vi "Update Connection.vi"(8 "error in (no error)":errorcluster, 10 "Connection Info":T1, 11 "VectoService in":refnum<class "VectoInfo.lvclass">) -> (0 "error out":errorcluster, 3 "VectoService out":refnum<class "VectoInfo.lvclass">)   [LabVIEW 2020, in "Vecto.lvlib" / "VectoInfo.lvclass"]
uses:
  VectoInfo.lvclass
  Connection Info.ctl
  Connection Type.ctl
  Connection Data.ctl
  VectoInfo.lvclass/VectoInfo.ctl
  Vecto.lvlib
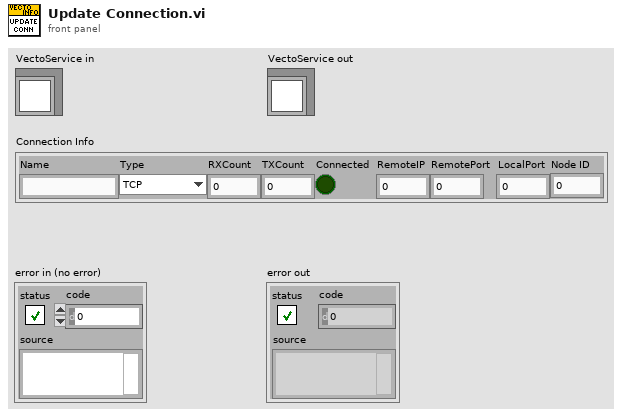
[diagram p1: front panel]
types:
  T1 = typedef "Vecto.lvlib/Connection Info.ctl" = cluster{"Name":string, "Type":T2, "RXCount":i32, "TXCount":i32, "Connected":bool, "RemoteIP":u32, "RemotePort":u16, "LocalPort":u16, "Node ID":u32}
  T2 = typedef "Vecto.lvlib/Connection Type.ctl" = enum16{"TCP", "Telemetry", "Discovery", "HTTP"}
  T3 = typedef "Vecto.lvlib/VectoInfo.lvclass/Connection Data.ctl" = cluster{"Info":T1}
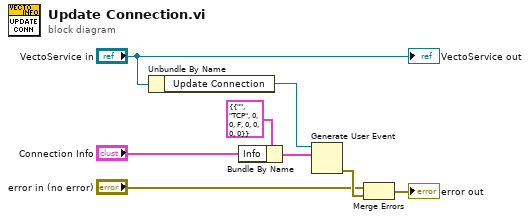
[diagram p0: block diagram]
diagram:
  n1 = Unbundle By Name("VectoService in") -> ("Update Connection"=w8:refnum<user-event>)
  n2 = Bundle By Name(cluster=T3 {"Info"={"Name"="", "Type"=enum."TCP", "RXCount"=0, "TXCount"=0, "Connected"=FALSE, "RemoteIP"=0, "RemotePort"=0, "LocalPort"=0, "Node ID"=0}} ("event data"), "Info"="Connection Info") -> (w6:T3)
  n3 = Generate User Event(user event=w8, event data cluster=w6) -> (error out=w3:errorcluster)  [unwired: 2 in, 1 out]
  n4 = Merge Errors("error in (no error)", w3) -> (→"error out":errorcluster)
  "VectoService out" <- "VectoService in"
